vi "Teleop.vi"(0 "error in":errorcluster, 2 "Twist":T1, 3 "node":string) -> (1 "error out":errorcluster)   [LabVIEW 2015]
doc: "Writes to the Turtlebot's topic teleop"
uses:
  ROS/Code/Console/Servers/ServerSubs/TopicDef.ctl
  ROS/Code/SubVIs/_ROSDirection.ctl
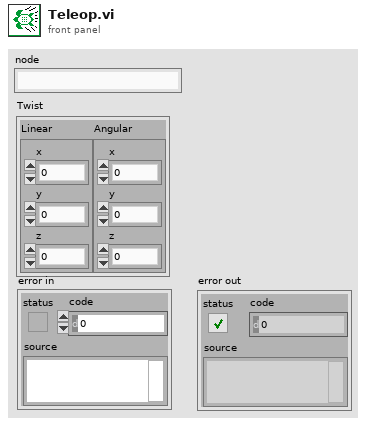
[diagram p1: front panel]
types:
  T1 = cluster{"Linear":cluster{"x":dbl, "y":dbl, "z":dbl}, "Angular":cluster{"x":dbl, "y":dbl, "z":dbl}}
  T2 = typedef "TopicDef.ctl" = cluster{"Topic":string, "Type":string, "Action":T3, "Update (ms)":u16, "queue size":u16}
  T3 = typedef "_ROSDirection.ctl" = enum16{"Node", "Publisher", "Subscriber", "ServiceClient", "ServiceProvider"}
  T4 = typedef "_ROSControl.ctl" = cluster{"topic port":u16, "Node":string, "topic":string, "type":string, "node port":u16, "error ":errorcluster, "Direction":T3, "Update (ms)":u16, "FIFO size":u16}
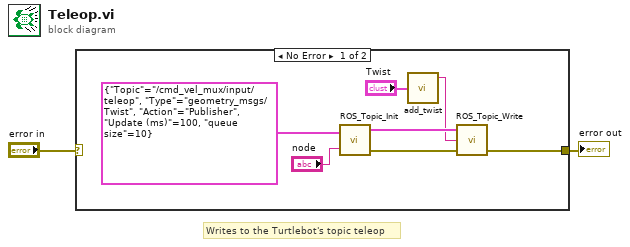
[diagram p0: block diagram]
diagram:
  # "Writes to the Turtlebot's topic teleop"
  n1 = case shown="No Error" "error in" {
    selector: "error in" -> [_ w10]
    tunnel: [w4 w10] -> w1
    frame No Error {
      n2 = call "ROS_Topic_Init.vi"("Definitions"=T2 {"Topic"="/cmd_vel_mux/input/teleop", "Type"="geometry_msgs/Twist", "Action"=enum."Publisher", "Update (ms)"=100, "queue size"=10}, "node"="node") -> ("ROS out"=w8:T4, "error out"=w7:errorcluster)  [unwired: 1 in]
      n3 = call "add_twist.vi"("Twist"="Twist") -> ("msg out"=w6:string)  [unwired: 4 in]
      n4 = call "ROS_Topic_Write.vi"("error in (no error)"=w7, "Msg in"=w6, "ROS in"=w8) -> ("error out"=w4:errorcluster)  [unwired: 1 in, 1 out]
    }
    frame Error {
    }
  }
  "error out" <- w1
